vi "PSNR(dB).vi"(10 "Image Pixels (Float) 2":dbl[][](array[numeric]), 11 "Image Pixels (Float) 1":dbl[][](array[numeric])) -> (0 "min diff":dbl, 1 "max diff":dbl, 2 "Mean Square Error (MSE)":dbl, 3 "PSNR (dB)":dbl, 4 "Difference":sgl[][](array[numeric]))   [LabVIEW 2023]
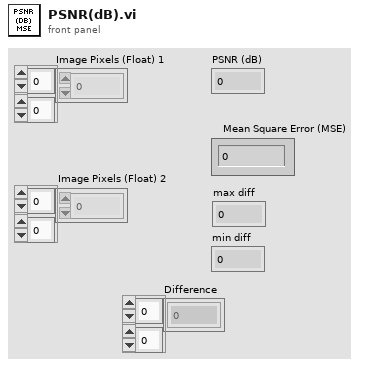
[diagram p1: front panel]
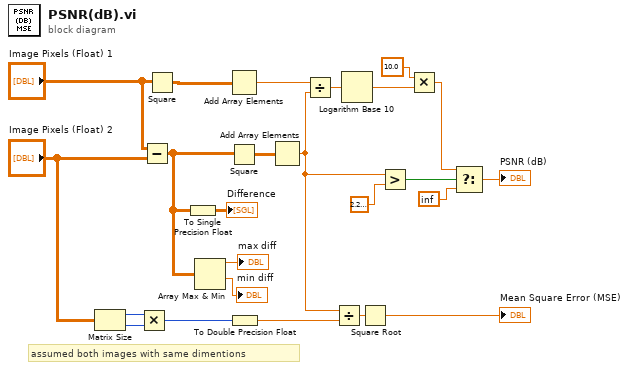
[diagram p0: block diagram]
diagram:
  # "assumed both images with same dimentions"
  n1 = Matrix Size(0:"Image Pixels (Float) 2") -> (1:w12:i32, 2:w11:i32)
  n2 = Multiply(x=w12, y=w11) -> (x*y=w10:i32)
  n3 = Subtract(x="Image Pixels (Float) 1", y="Image Pixels (Float) 2") -> (x-y=w3:dbl[][])
  n4 = Square(x="Image Pixels (Float) 1") -> (x^2=w21:dbl[][])
  n5 = To Single Precision Float(number=w3) -> (single precision float=→"Difference":sgl[][])
  n6 = Array Max & Min(array=w3) -> (max value=→"max diff":dbl, min value=→"min diff":dbl)  [unwired: 2 out]
  n7 = Add Array Elements(numeric array=w21) -> (sum=w7:dbl)
  n8 = Square(x=w3) -> (x^2=w20:dbl[][])
  n9 = To Double Precision Float(number=w10) -> (double precision float=w5:dbl)
  n10 = Add Array Elements(numeric array=w20) -> (sum=w6:dbl)
  n11 = Divide(x=w7, y=w6) -> (x/y=w22:dbl)
  n12 = Divide(x=w6, y=w5) -> (x/y=w13:dbl)
  n13 = Logarithm Base 10(1:w22) -> (0:w23:dbl)
  n14 = Square Root(x=w13) -> (sqrt(x)=→"Mean Square Error (MSE)":dbl)
  n15 = Greater?(x=w6, y=2.220446049250313e-16) -> (0:w18:bool)
  n16 = Multiply(x=10.0, y=w23) -> (x*y=w17:dbl)
  n17 = Select(t=w17, s=w18, f=inf) -> (s? t:f=→"PSNR (dB)":dbl)
